vi "OP600ZP_ISO.vi"(8 "entrée d'erreur (pas d'erreur)":errorcluster, 9 "Oui":bool, 10 "reference en entrée":refnum<vi>) -> (0 "sortie d'erreur":errorcluster, 1 "ISOM":string, 2 "ISOP":string, 3 "Booléen":bool)   [LabVIEW 2020]
uses:
  VG/PackType.vi
  OP600ZP_VGConf.vi
panel:
  out "BDD":T1
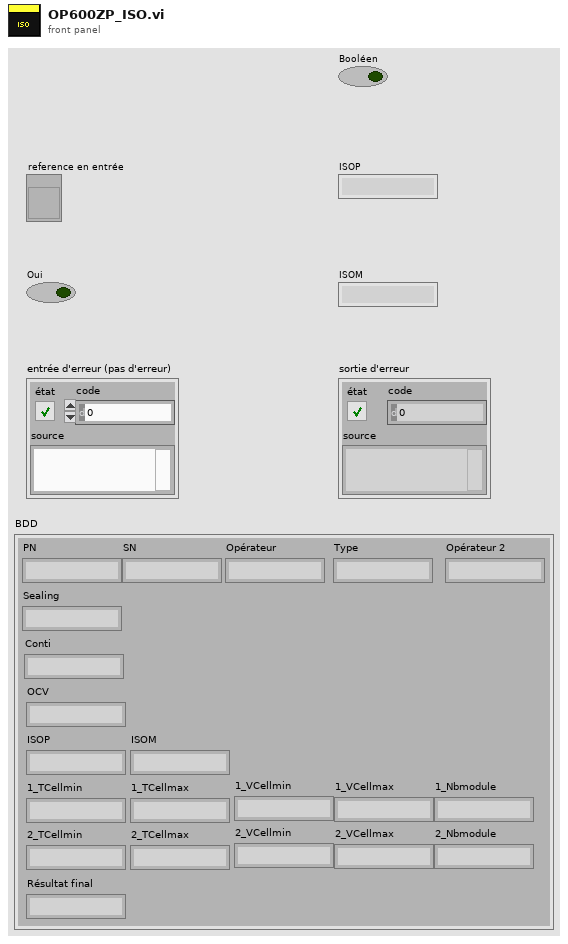
[diagram p1: front panel]
types:
  T1 = cluster{"PN":string, "Opérateur":string, "Sealing":string, "Conti":string, "OCV":string, "ISOP":string, "ISOM":string, "1_TCellmin":string, "1_TCellmax":string, "1_VCellmin":string, "1_VCellmax":string, "1_Nbmodule":string, "2_TCellmin":string, "2_TCellmax":string, "2_VCellmin":string, "2_VCellmax":string, "2_Nbmodule":string, "Résultat final":string, "Type":string, "Opérateur 2":string, "SN":string}
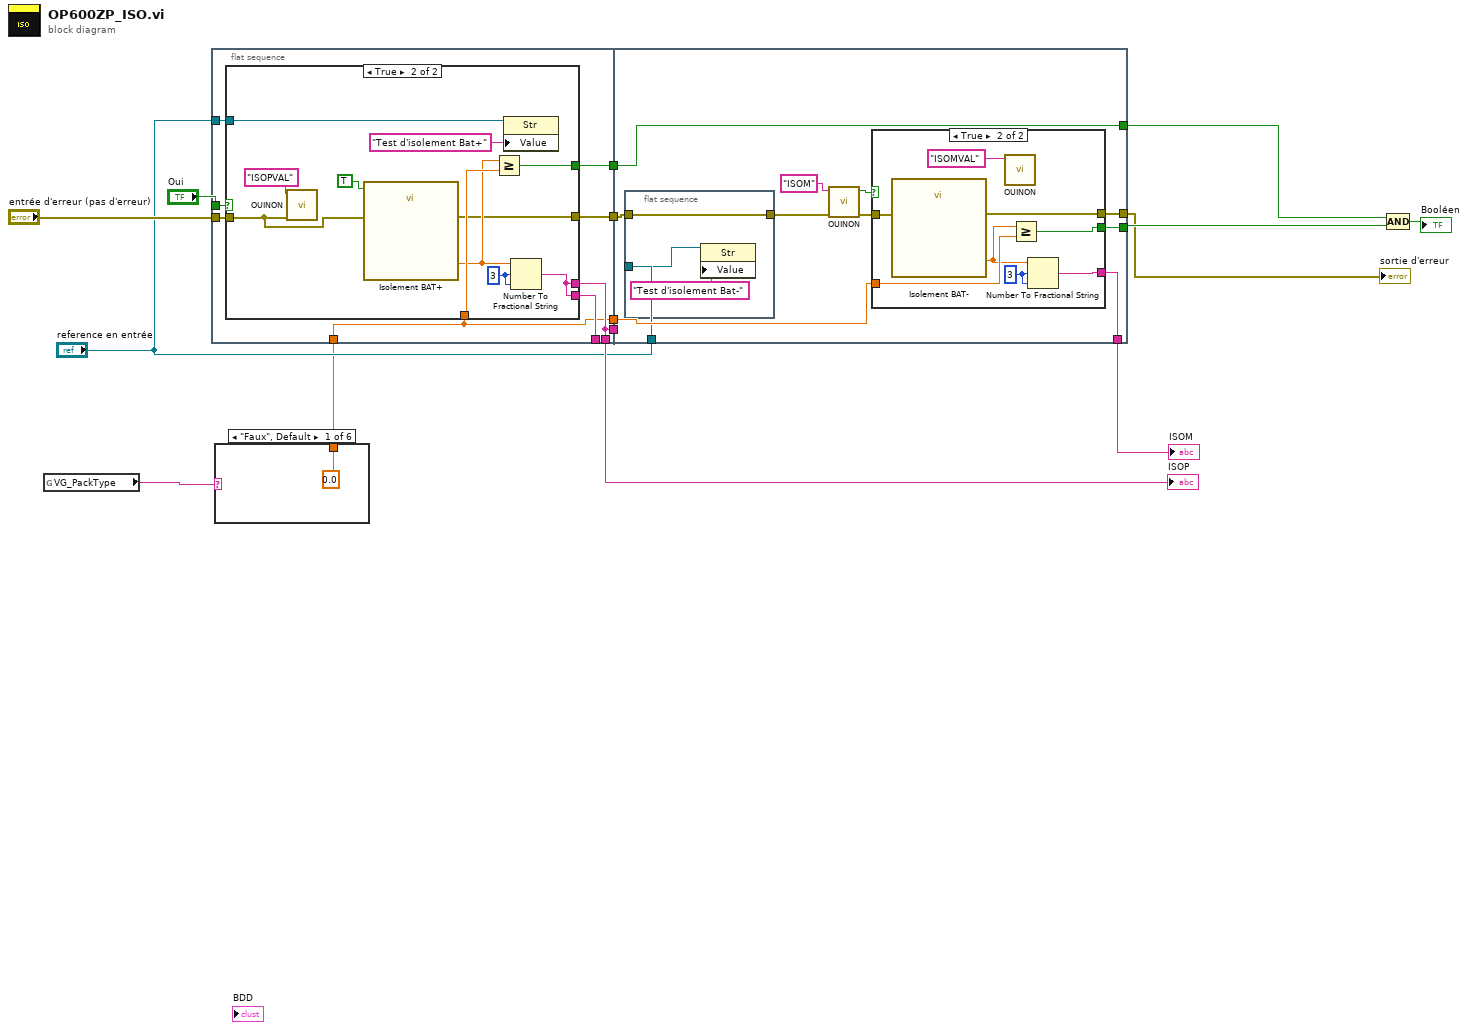
[diagram p0: block diagram]
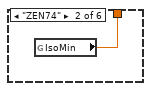
[diagram p2: hidden frame]
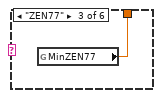
[diagram p3: hidden frame]
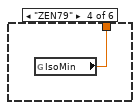
[diagram p4: hidden frame]
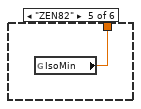
[diagram p5: hidden frame]
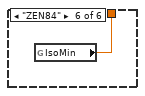
[diagram p6: hidden frame]
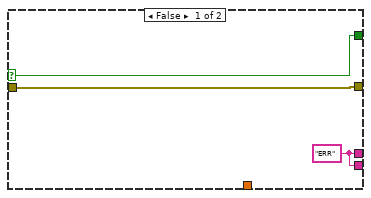
[diagram p7: hidden frame]
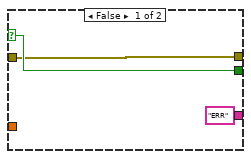
[diagram p8: hidden frame]
diagram:
  n1 = global read "PackType.vi" "VG_PackType"() -> (w3:string)
  n2 = flat-sequence {
    tunnel: [w23] -> _
    tunnel: [w16] -> w15
    tunnel: [w20] -> w14
    tunnel: [w22] -> w13
    tunnel: [w21] -> w12
    tunnel: [w20] -> w9
    tunnel: "entrée d'erreur (pas d'erreur)" -> [w19]
    tunnel: "Oui" -> [w18]
    tunnel: "reference en entrée" -> [w17]
    tunnel: w2 -> [w16]
    tunnel: w15 -> [w43]
    tunnel: w14 -> [_]
    tunnel: w13 -> [w48]
    tunnel: w12 -> [w47]
    tunnel: [w41] -> w8
    tunnel: "reference en entrée" -> [w39]
    tunnel: [w48] -> w5
    tunnel: [w42] -> w7
    tunnel: [w38] -> w1
    frame #0 {
      n3 = case shown="True" w18 {
        selector: w18 -> [w25 _]
        tunnel: w19 -> [w26 w27]
        tunnel: [w26 w30] -> w21
        tunnel: [w24 w33] -> w20
        tunnel: [w25 w34] -> w22
        tunnel: w16 -> [_ w36]
        tunnel: [w24 w33] -> w23
        tunnel: w17 -> [_ w28]
        frame False {
          w24 = "ERR"
        }
        frame True {
          w37 = i16 3 ("largeur (-)")
          n4 = call "OUINON.vi"("errin"=w27, "image"="ISOPVAL") -> ()  [unwired: 8 in, 2 out]
          n5 = call "Isolement BAT+"("Enable"=TRUE, "error in (no error)"=w27) -> ("ISOP"=w35:dbl, "error out"=w30:errorcluster)  [unwired: 15 in, 1 out]
          n6 = Greater Or Equal?(x=w35, y=w36) -> (x >= y?=w34:bool)
          n7 = property class="Str"(reference=w28, "Value"="Test d'isolement Bat+" ("TOP")) -> ()  [unwired: 1 in, 2 out]
          n8 = Number To Fractional String(number=w35, width (-)=w37, precision (6)=w37) -> (F-format string=w33:string)  [unwired: 1 in]
        }
      }
    }
    frame #1 {
      n9 = flat-sequence {
        tunnel: w47 -> [w50]
        tunnel: [w50] -> w46
        tunnel: w39 -> [w49]
        frame #0 {
          n10 = property class="Str"(reference=w49, "Value"="Test d'isolement Bat-" ("TOP")) -> ()  [unwired: 1 in, 2 out]
        }
      }
      n11 = call "OUINON.vi"("errin"=w46, "image"="ISOM" ("IN")) -> ("error out"=w40:errorcluster, "OUI/NON"=w44:bool)  [unwired: 8 in]
      n12 = case shown="True" w44 {
        selector: w44 -> [w54 _]
        tunnel: [w52 w58] -> w38
        tunnel: ["ERR" w57] -> w41
        tunnel: [w54 w59] -> w42
        tunnel: w43 -> [_ w61]
        tunnel: w40 -> [w52 w55]
        frame False {
        }
        frame True {
          w62 = i16 3 ("largeur (-)")
          n13 = call "Isolement BAT-"("error in (no error)"=w55) -> ("ISOM"=w60:dbl, "error out"=w58:errorcluster)  [unwired: 16 in, 1 out]
          n14 = call "OUINON.vi"("image"="ISOMVAL") -> ()  [unwired: 9 in, 2 out]
          n15 = Greater Or Equal?(x=w60, y=w61) -> (x >= y?=w59:bool)
          n16 = Number To Fractional String(number=w60, width (-)=w62, precision (6)=w62) -> (F-format string=w57:string)  [unwired: 1 in]
        }
      }
    }
  }
  n17 = case shown="\"Faux\", Default" w3 {
    tunnel: [0.0 ("IsoMin") w64 w65 w66 w67 w68] -> w2
    frame "Faux", Default {
    }
    frame "ZEN74" {
      n18 = global read "OP600ZP_VGConf.vi" "IsoMin"() -> (w64:dbl)
    }
    frame "ZEN77" {
      n19 = global read "OP600ZP_VGConf.vi" "MinZEN77"() -> (w65:dbl)
    }
    frame "ZEN79" {
      n20 = global read "OP600ZP_VGConf.vi" "IsoMin"() -> (w66:dbl)
    }
    frame "ZEN82" {
      n21 = global read "OP600ZP_VGConf.vi" "IsoMin"() -> (w67:dbl)
    }
    frame "ZEN84" {
      n22 = global read "OP600ZP_VGConf.vi" "IsoMin"() -> (w68:dbl)
    }
  }
  n23 = Compound Arithmetic op=AND ("Opérateur arithmétique")(w5, w7) -> (→"Booléen":bool)
  "ISOP" <- w9
  "ISOM" <- w8
  "sortie d'erreur" <- w1
